vi "PDO unlink DSP402.vi"(4 "error in (no error)":errorcluster, 5 "Indices":cluster{"Communication":u32, "Mapping":u32}={"Communication"=6144, "Mapping"=6656} {"Mapping" format="%x"; "Communication" format="%x"}, 6 "Cob ID":u32, 7 "DSP402 in":refnum<class "DSP402.lvclass">) -> (0 "error out":errorcluster, 3 "DSP402 out":refnum<class "DSP402.lvclass">)   [LabVIEW 2026, in "canopen_.lvlib" / "DSP402.lvclass"]
uses:
  DSP402.lvclass
  DSP402.lvclass/DSP402.ctl
  CANopen/CANopen.lvclass
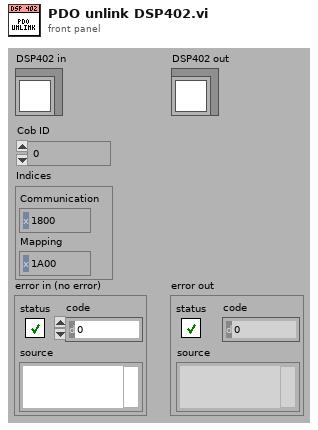
[diagram p1: front panel]
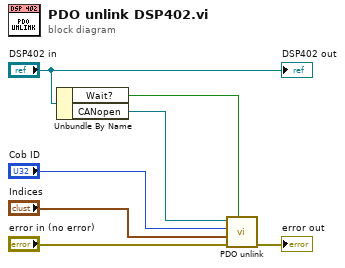
[diagram p0: block diagram]
diagram:
  n1 = Unbundle By Name("DSP402 in") -> ("Wait?"=w4:bool, "CANopen"=w3:refnum<class "CANopen.lvclass">)
  n2 = call "PDO unlink.vi"("Wait?"=w4, "error in (no error)"="error in (no error)", "Indices"="Indices", "Cob ID"="Cob ID", "CANopen in"=w3) -> ("error out"=→"error out":errorcluster)  [unwired: 1 in, 2 out]
  "DSP402 out" <- "DSP402 in"
